vi "Write Data.vi"(7 "UART":refnum<class "UART.lvclass">, 8 "error in (no error)":errorcluster, 10 "Data":string, 11 "Session In":refnum<class "Session.lvclass">) -> (0 "error out":errorcluster, 3 "Session Out":refnum<class "Session.lvclass">)   [LabVIEW 2020, in "CTI.lvlib" / "UART.lvclass"]
uses:
  UART.lvclass/UART.ctl
  UART.lvclass
  Session/Session.lvclass
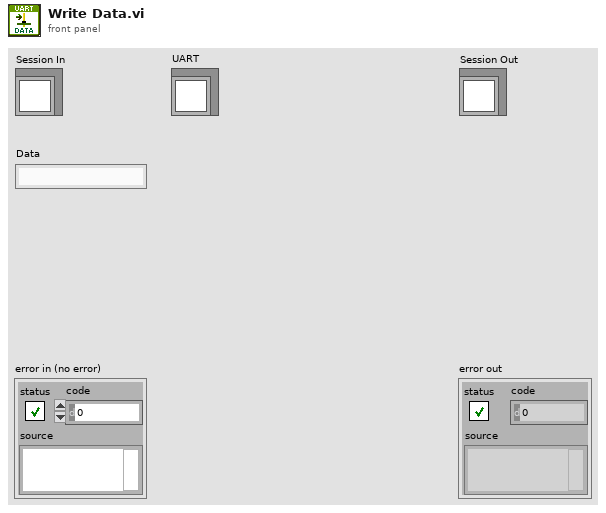
[diagram p1: front panel]
types:
  T1 = typedef "CTI.lvlib/UART Number.ctl" = i8
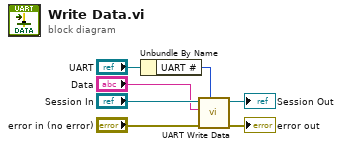
[diagram p0: block diagram]
diagram:
  n1 = Unbundle By Name("UART") -> ("UART #"=w2:T1)
  n2 = call-dynamic "UART Write Data.vi"("UART #"=w2, "error in (no error)"="error in (no error)", "Data"="Data", "Session in"="Session In") -> ("error out"=→"error out":errorcluster, "Session out"=→"Session Out":refnum<class "Session.lvclass">)  [unwired: 6 in]
